vi "RSZVB Set IMOD Lower Tone Source.vi"(7 "Source Number (1)":i32=1, 8 "error in (no error)":errorcluster {"code" format="%.0x"}, 9 "Source (0: Port)":i32(ring) items=["Port", "Generator"], 10 "Channel (1)":i32=1, 11 "VISA session":refnum<visa-resource-name>) -> (0 "error out":errorcluster {"code" format="%.0x"}, 3 "dup VISA session":refnum<visa-resource-name>)   [LabVIEW 2011]
doc: "This VI selects the source for the lower tone signal that is used for the intermodulation measurement.\n\nNote(s):\n\n(1) This VI is not available for R&S ZVB instrument.\n\nRemote-control command(s):\n[SENSe<Ch>:]FREQuency:IMODulation:LTONe NONE | PORT | GENerator, <source_no>"
uses:
  _utility/RSZVB Global Data.vi
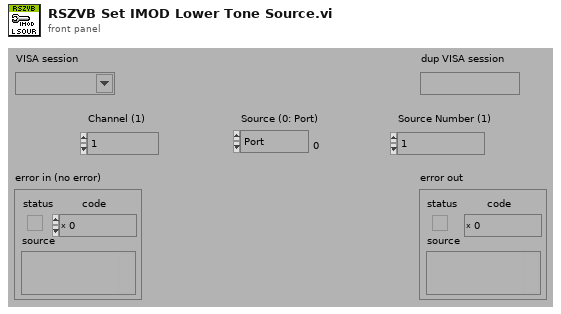
[diagram p1: front panel]
types:
  T1 = cluster{"Error Checking (T: On)":bool, "Installed Options":string[], "Data Valid?":bool, "Ports":i32, "Model":string[], "Option Checking (T: On)":bool}[]
  T2 = cluster{"Error Checking (T: On)":bool, "Installed Options":string[], "Data Valid?":bool, "Ports":i32, "Model":string[], "Option Checking (T: On)":bool}
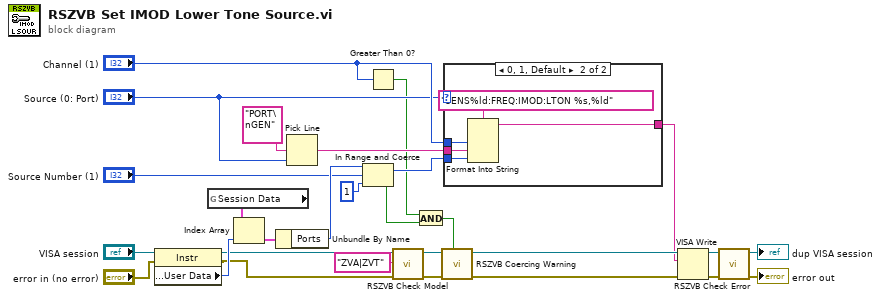
[diagram p0: block diagram]
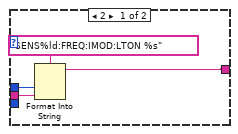
[diagram p2: hidden frame]
diagram:
  n1 = property class="Instr"(reference="VISA session", error in="error in (no error)") -> (reference out=w3:refnum<visa-resource-name>, error out=w2:errorcluster, "General Settings:User Data"=w28:u32)
  n2 = global read "RSZVB Global Data.vi" "Session Data"() -> (w27:T1)
  n3 = Index Array(array=w27, index=w28) -> (element=w26:T2)
  n4 = Unbundle By Name(w26) -> ("Ports"=w16:i32)
  n5 = Pick Line(multi-line string="PORT\nGEN", line index="Source (0: Port)") -> (output string=w19:string)  [unwired: 1 in]
  n6 = In Range and Coerce(upper limit=w16, x="Source Number (1)", lower limit=1) -> (coerced(x)=w12:i32, In Range?=w11:bool)
  n7 = Greater Than 0?(x="Channel (1)") -> (x > 0?=w10:bool)
  n8 = call "RSZVB Check Model.vi"("error in (no error)"=w2, "Model"="ZVA|ZVT", "VISA session"=w3) -> ("error out"=w5:errorcluster, "dup VISA session"=w4:refnum<visa-resource-name>)  [unwired: 7 in]
  n9 = And(x=w10, y=w11) -> (x .and. y?=w9:bool)
  n10 = call "RSZVB Coercing Warning.vi"("In Range?"=w9, "error in (no error)"=w5, "VISA session"=w4) -> ("error out"=w23:errorcluster, "dup VISA session"=w22:refnum<visa-resource-name>)  [unwired: 7 in]
  n11 = case shown="0, 1, Default" "Source (0: Port)" {
    tunnel: "Channel (1)" -> [w31 w36]
    tunnel: w19 -> [w30 w35]
    tunnel: w12 -> [_ w34]
    tunnel: [w29 w33] -> w8
    frame 2 {
      n12 = Format Into String(format string="SENS%ld:FREQ:IMOD:LTON %s", w31, w30) -> (resulting string=w29:string)  [unwired: 2 in, 1 out]
    }
    frame 0, 1, Default {
      n13 = Format Into String(format string="SENS%ld:FREQ:IMOD:LTON %s,%ld", w36, w35, w34) -> (resulting string=w33:string)  [unwired: 2 in, 1 out]
    }
  }
  n14 = VISA Write(VISA resource name=w22, write buffer=w8, error in (no error)=w23) -> (VISA resource name out=w25:refnum<visa-resource-name>, error out=w24:errorcluster)  [unwired: 1 out]
  n15 = call "RSZVB Check Error.vi"("error in (no error)"=w24, "VISA session"=w25) -> ("error out"=→"error out":errorcluster, "dup VISA session"=→"dup VISA session":refnum<visa-resource-name>)  [unwired: 8 in]
